vi "stimulator.vi"(11 "Boolean 2":bool) -> ()   [LabVIEW 2009]
uses:
  <vilib>/DAQmx/write.llb/DAQmx Write (Digital Bool 1Line 1Point).vi
panel:
  in  "stop":bool
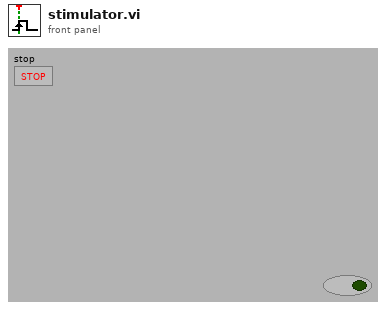
[diagram p1: front panel]
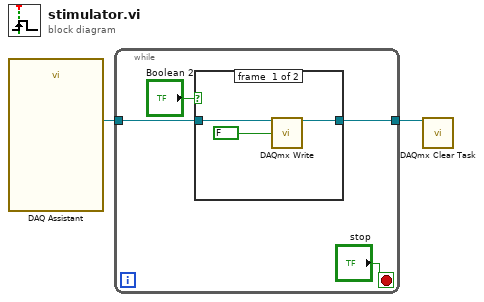
[diagram p0: block diagram]
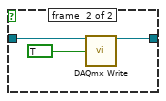
[diagram p2: hidden frame]
diagram:
  n1 = call "DAQ Assistant"() -> ("task out"=w2:refnum<k21>)  [unwired: 18 in, 1 out]
  n2 = while {
    tunnel: w2 -> [w6]
    tunnel: [w5] -> w1
    stop <- "stop" stop-if-true
    n3 = case shown="True" "Boolean 2" {
      tunnel: w6 -> [w8 w12]
      tunnel: [w7 w10] -> w5
      frame #0 {
        n4 = call-poly <vilib>:"DAQmx Write.vi"("task/channels in"=w8, "data"=FALSE) -> ("task out"=w7:refnum<k21>)  [unwired: 11 in, 2 out]
      }
      frame #1 {
        n5 = call-poly <vilib>:"DAQmx Write.vi"("task/channels in"=w12, "data"=TRUE) -> ("task out"=w10:refnum<k21>)  [unwired: 11 in, 2 out]
      }
    }
  }
  n6 = call <vilib>:"DAQmx Clear Task.vi"("task in"=w1) -> ()  [unwired: 14 in, 1 out]
